vi "Save_scan_as_BMP_sub_vi.vi"(8 "error in (no error)":errorcluster, 9 "NID Path In":string, 10 "Application":refnum<k7>, 11 "BMP Path In":path) -> (0 "Error Out":errorcluster, 2 "BMP":picture, 3 "BMP Path Out":path)   [LabVIEW 2016]
uses:
  <vilib>/picture/picture.llb/imagedata.ctl
panel:
  out "IsObj":bool
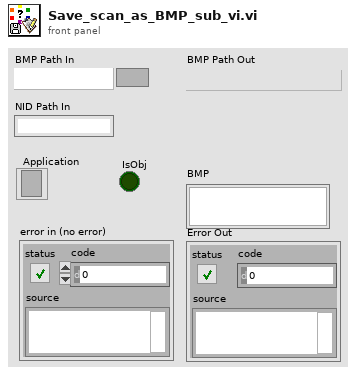
[diagram p1: front panel]
types:
  T1 = cluster{"left":i16, "top":i16, "right":i16, "bottom":i16}
  T2 = typedef "imagedata.ctl" = cluster{"image type":i32, "image depth":i32, "image":u8[], "mask":u8[], "colors":u32[], "Rectangle":cluster{"left":i16, "top":i16, "right":i16, "bottom":i16}}
  T3 = typedef "LVRectTypeDef.ctl" = cluster{"Left":i16, "Top":i16, "Right":i16, "Bottom":i16}
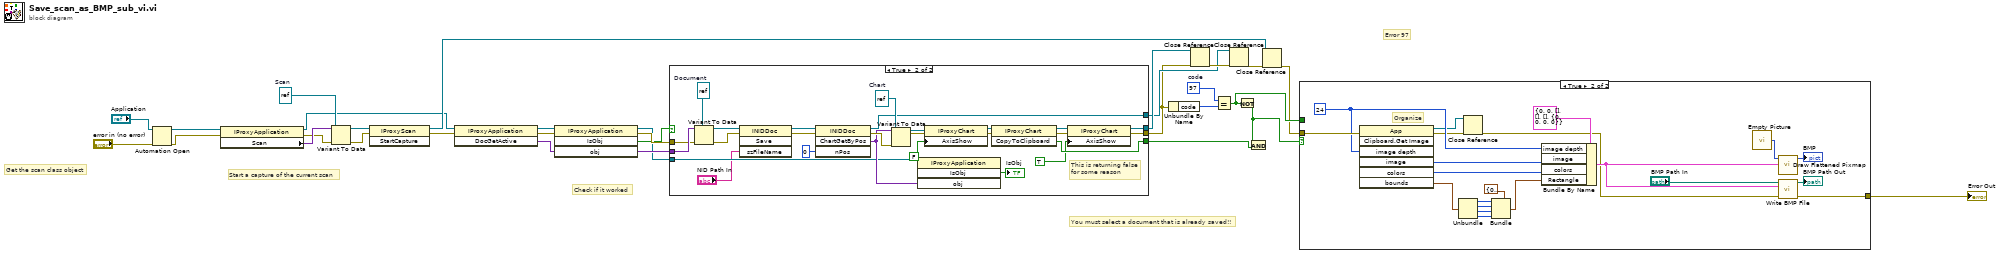
[diagram p0: block diagram]
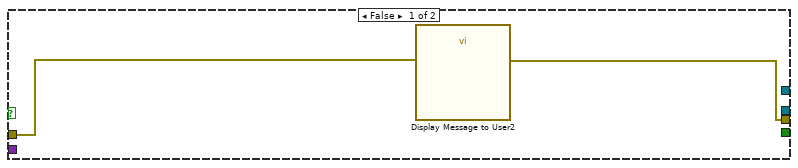
[diagram p2: hidden frame]
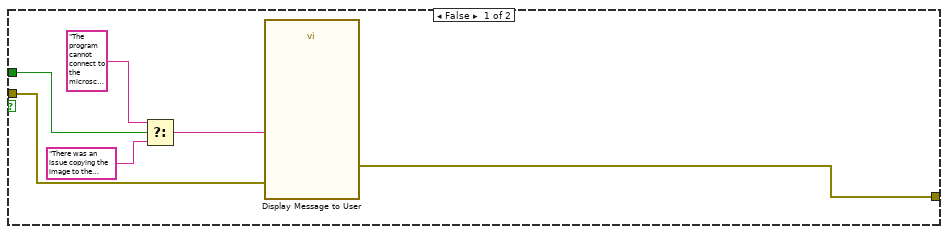
[diagram p3: hidden frame]
diagram:
  w11 = refnum<k7> refnum  # Scan
  w27 = 97  # code
  # "Check if it worked"
  # "Start a capture of the current scan"
  # "Get the scan class object"
  # "You must select a document that is already saved!!"
  # "Error 97"
  n1 = Automation Open(error in (no error)="error in (no error)", Automation Refnum="Application") -> (Automation Refnum=w14:refnum<k7>, error out=w13:errorcluster)  [unwired: 2 in]
  n2 = property class="IProxyApplication"(reference=w14, error in=w13) -> (reference out=w7:refnum<k7>, error out=w6:errorcluster, "Scan"=w17:variant)
  n3 = Variant To Data(error in=w6, type=w11, Variant=w17) -> (data=w16:refnum<k7>, error out=w15:errorcluster)
  n4 = invoke class="IProxyScan" method="StartCapture"(reference=w16, error in=w15) -> (reference out=w9:refnum<k7>, error out=w12:errorcluster)  [unwired: 1 in, 1 out]
  n5 = invoke class="IProxyApplication" method="DocGetActive"(reference=w7, error in=w12) -> (reference out=w31:refnum<k7>, error out=w28:errorcluster, "DocGetActive"=w21:variant)  [unwired: 1 in]
  n6 = invoke class="IProxyApplication" method="IsObj"(reference=w31, error in=w28, "obj"=w21) -> (reference out=w5:refnum<k7>, error out=w29:errorcluster, "IsObj"=w4:bool, "obj"=w30:variant)  [unwired: 1 in]
  n7 = case shown="True" w4 {
    tunnel: [_ w46] -> w25
    tunnel: w30 -> [_ w58]
    tunnel: w29 -> [w32 w57]
    tunnel: [w33 w47] -> w1
    tunnel: [_ w44] -> w20
    tunnel: [_ w43] -> w3
    tunnel: w5 -> [_ w40]
    frame False {
      n8 = call "Display Message to User2"("error in (no error)"=w32) -> ("error out"=w33:errorcluster)  [unwired: 9 in, 1 out]
    }
    frame True {
      w59 = refnum<k7> refnum  # Document
      w50 = refnum<k7> refnum  # Chart
      # "This is returning false\nfor some reason"
      n9 = Variant To Data(error in=w57, type=w59, Variant=w58) -> (data=w38:refnum<k7>, error out=w36:errorcluster)
      n10 = invoke class="INIDDoc" method="Save"(reference=w38, error in=w36, "szFileName"="NID Path In") -> (reference out=w37:refnum<k7>, error out=w35:errorcluster)  [unwired: 1 in, 2 out]
      n11 = invoke class="INIDDoc" method="ChartGetByPos"(reference=w37, error in=w35, "nPos"=0) -> (reference out=w43:refnum<k7>, error out=w56:errorcluster, "ChartGetByPos"=w42:variant)  [unwired: 1 in, 1 out]
      n12 = Variant To Data(error in=w56, type=w50, Variant=w42) -> (data=w55:refnum<k7>, error out=w52:errorcluster)
      n13 = invoke class="IProxyApplication" method="IsObj"(reference=w40, "obj"=w42) -> ("IsObj"=→"IsObj":bool)  [unwired: 2 in, 3 out]
      n14 = property class="IProxyChart"(reference=w55, error in=w52, "AxisShow"=FALSE) -> (reference out=w53:refnum<k7>, error out=w51:errorcluster)
      n15 = invoke class="IProxyChart" method="CopyToClipboard"(reference=w53, error in=w51) -> (reference out=w49:refnum<k7>, error out=w48:errorcluster, "CopyToClipboard"=w46:bool)  [unwired: 1 in]
      n16 = property class="IProxyChart"(reference=w49, error in=w48, "AxisShow"=TRUE) -> (reference out=w44:refnum<k7>, error out=w47:errorcluster)
    }
  }
  n17 = Unbundle By Name(w1) -> ("code"=w26:i32)
  n18 = Close Reference(reference=w20, error in (no error)=w1) -> (error out=w19:errorcluster)
  n19 = Equal?(x=w27, y=w26) -> (x = y?=w24:bool)
  n20 = Close Reference(reference=w3, error in (no error)=w19) -> (error out=w8:errorcluster)
  n21 = Not(x=w24) -> (.not. x?=w18:bool)
  n22 = And(x=w18, y=w25) -> ()  [unwired: 1 out]
  n23 = Close Reference(reference=w9, error in (no error)=w8) -> (error out=w2:errorcluster)
  n24 = case shown="True" w18 {
    tunnel: w2 -> [w65 w86]
    tunnel: w24 -> [w64 _]
    tunnel: [w60 w71] -> w23
    frame False {
      n25 = Select(t="The program cannot connect to the microscope API, please make sure to view the Access Codes before using the program.  If the program still does not work, then try exiting the control software, and then using  task manager to close out of the program fully.", s=w64, f="There was an issue copying the image to the clipboard, please export image manually. ") -> (s? t:f=w61:string)
      n26 = call "Display Message to User"("error in (no error)"=w65, "Message"=w61) -> ("error out"=w60:errorcluster)  [unwired: 8 in, 1 out]
    }
    frame True {
      w73 = 24 ("Image Depth")
      # "Organize"
      n27 = invoke class="App" method="Clipboard.Get Image"(error in=w86, "image depth"=w73) -> (reference out=w66:refnum<vi>, error out=w68:errorcluster, "image"=w85:u8[], "colors"=w84:u32[], "bounds"=w76:T3)  [unwired: 5 in, 2 out]
      n28 = Unbundle(w76) -> ("Left"=w80:i16, "Top"=w79:i16, "Right"=w78:i16, "Bottom"=w77:i16)
      n29 = Close Reference(reference=w66, error in (no error)=w68) -> (error out=w67:errorcluster)
      n30 = Bundle(cluster=T1 {"left"=0, "top"=0, "right"=0, "bottom"=0} ("Rectangle"), "left"=w80, "top"=w79, "right"=w78, "bottom"=w77) -> (w75:T1)
      n31 = Bundle By Name(cluster=T2 {"image type"=0, "image depth"=0, "image"=[], "mask"=[], "colors"=[], "Rectangle"={"left"=0, "top"=0, "right"=0, "bottom"=0}} ("image data"), "image depth"=w73, "image"=w85, "colors"=w84, "Rectangle"=w75) -> (w74:T2)
      n32 = call "Empty Picture"() -> ("empty picture"=w83:picture)
      n33 = call <vilib>:"Draw Flattened Pixmap.vi"("image data"=w74, "picture"=w83) -> ("new picture"=→"BMP":picture)  [unwired: 7 in]
      n34 = call <vilib>:"Write BMP File.vi"("error in (no error)"=w67, "image data"=w74, "path to BMP file"="BMP Path In") -> ("error out"=w71:errorcluster, "path"=→"BMP Path Out":path)  [unwired: 7 in]
    }
  }
  "Error Out" <- w23
